vi "LDA_Dimensions.vi"(11 "LDA set up":T1) -> (3 "Numeric":i32)   [LabVIEW 2018]
uses:
  Controls/LDA_Setup.ctl
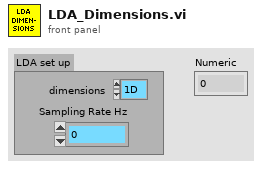
[diagram p1: front panel]
types:
  T1 = typedef "LDA_Setup.ctl" = cluster{"dimensions":enum16{"1D", "2D", "3D", "4D", "5D"}, "Sampling Rate Hz":dbl}
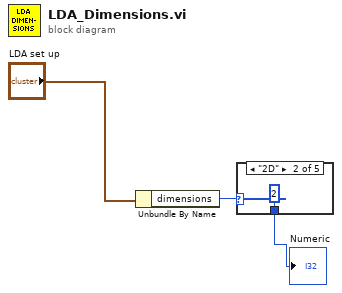
[diagram p0: block diagram]
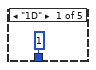
[diagram p2: hidden frame]
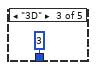
[diagram p3: hidden frame]
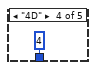
[diagram p4: hidden frame]
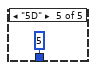
[diagram p5: hidden frame]
diagram:
  n1 = Unbundle By Name("LDA set up") -> ("dimensions"=w3:enum16{"1D", "2D", "3D", "4D", "5D"})
  n2 = case shown="\"2D\"" w3 {
    tunnel: [1 2 3 4 5] -> w1
    frame "1D" {
    }
    frame "2D" {
    }
    frame "3D" {
    }
    frame "4D" {
    }
    frame "5D" {
    }
  }
  "Numeric" <- w1
